vi "Abort Active DUT Airplane Mode Switching.vi"(8 "error in (no error)":errorcluster, 11 "VISA resource name":refnum<visa-resource-name>) -> (0 "error out":errorcluster, 3 "VISA resource name out":refnum<visa-resource-name>)   [LabVIEW 2015, in "Rohde&Schwarz CMXP Base.lvlib"]
doc: "Cancels switching the airplane mode at the DUT.\n\nAttribute:\nRSCMXPBASE_ATTR_ACTIVE_DUT_AIRPLANE_MODE_ABORT\n\nRemote-control command:\nABORt:DUT:CONTrol:AIRPlane"
uses:
  <instrlib>/Rohde&Schwarz CMXP Base/Rohde&Schwarz CMXP Base.lvlib
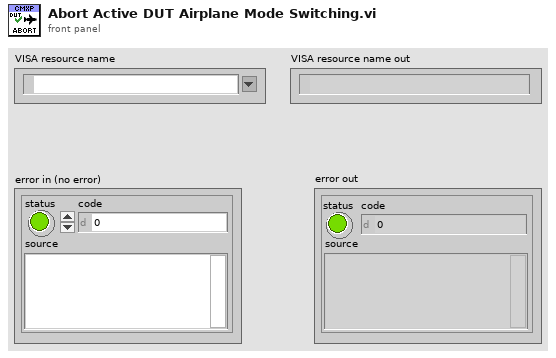
[diagram p1: front panel]
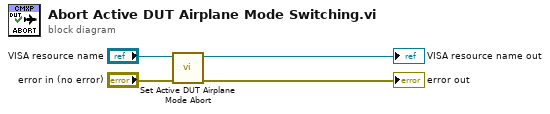
[diagram p0: block diagram]
diagram:
  n1 = call "Set Active DUT Airplane Mode Abort"("error in (no error)"="error in (no error)", "instrument handle"="VISA resource name") -> ("error out"=→"error out":errorcluster, "instrument handle out"=→"VISA resource name out":refnum<visa-resource-name>)  [unwired: 8 in]
